vi "Save Data.vi"(8 "error in (no error)":errorcluster, 10 "Numeric":dbl, 11 "Logging in":refnum<class "Logging.lvclass">) -> (0 "error out":errorcluster, 3 "Logging out":refnum<class "Logging.lvclass">)   [LabVIEW 2019, in "Logging.lvlib" / "Logging.lvclass"]
uses:
  Logging.lvclass
  Logging.lvclass/Logging.ctl
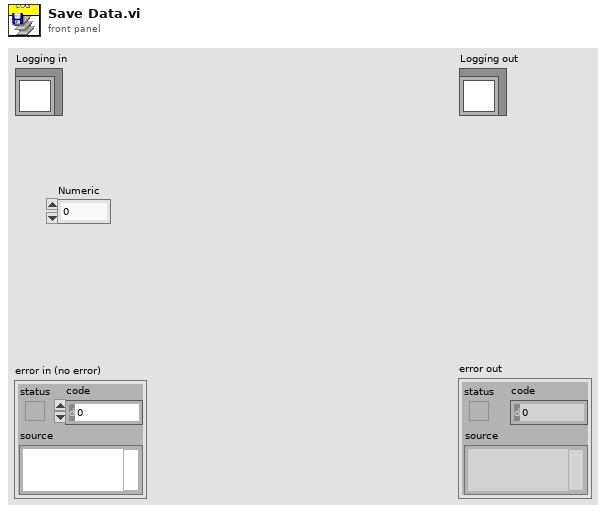
[diagram p1: front panel]
types:
  T1 = enum16{"open", "replace", "create", "open or create", "replace or create", "replace or create with confirmation"}
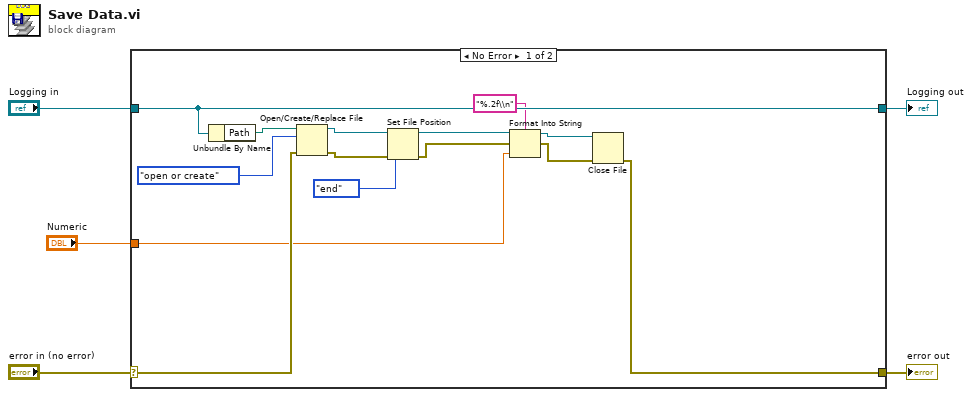
[diagram p0: block diagram]
diagram:
  n1 = case shown="No Error" "error in (no error)" {
    selector: "error in (no error)" -> [w14 w21]
    tunnel: [w13 w21] -> w4
    tunnel: [w19 w20] -> w2
    tunnel: "Logging in" -> [w19 w20]
    tunnel: "Numeric" -> [w6 _]
    frame No Error {
      n2 = Unbundle By Name(w19) -> ("Path"=w18:path)
      n3 = Open/Create/Replace File(file path (use dialog)=w18, error in=w14, operation (0:open)=T1."open or create") -> (refnum out=w12:refnum<file>, error out=w11:errorcluster)  [unwired: 3 in, 1 out]
      n4 = Set File Position(refnum=w12, from (0:start)=enum16{"start", "end", "current"}."end", error in=w11) -> (refnum out=w10:refnum<file>, error out=w9:errorcluster)  [unwired: 1 in]
      n5 = Format Into String(format string="%.2f\\n", initial string=w10, error in=w9, w6) -> (resulting string=w16:refnum<file>, error out=w15:errorcluster)
      n6 = Close File(refnum=w16, error in=w15) -> (error out=w13:errorcluster)  [unwired: 1 out]
    }
    frame Error {
    }
  }
  "error out" <- w4
  "Logging out" <- w2
